vi "CleanUp fp settings.vi"(4 "Original basic fp settings":T1, 5 "Front Panel Window:Panel Bounds":T2, 6 "error in (no error)":errorcluster, 9 "vi reference":refnum<vi>) -> (0 "error out":errorcluster, 3 "vi reference out":refnum<vi>)   [LabVIEW 2020]
uses:
  <vilib>/Utility/miscctls.llb/LVRectTypeDef.ctl
  Basic FP Settings--cluster.ctl
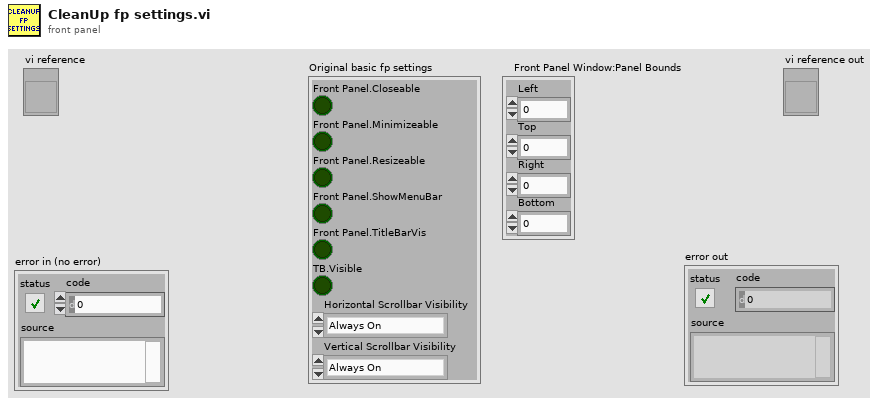
[diagram p1: front panel]
types:
  T1 = typedef "Basic FP Settings--cluster.ctl" = cluster{"Front Panel.Closeable":bool, "Front Panel.Minimizeable":bool, "Front Panel.Resizeable":bool, "Front Panel.ShowMenuBar":bool, "Front Panel.TitleBarVis":bool, "TB.Visible":bool, "Horizontal Scrollbar Visibility":enum16{"Always On", "Always Off", "Off While Running"}, "Vertical Scrollbar Visibility":enum16{"Always On", "Always Off", "Off While Running"}}
  T2 = typedef "LVRectTypeDef.ctl" = cluster{"Left":i16, "Top":i16, "Right":i16, "Bottom":i16}
  T3 = enum32{"Invalid", "Default", "Floating", "Floating/Auto-Hide", "Modal"}
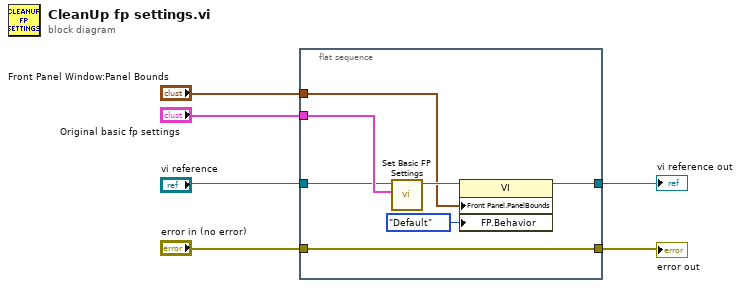
[diagram p0: block diagram]
diagram:
  n1 = flat-sequence {
    tunnel: "Original basic fp settings" -> [w11]
    tunnel: "Front Panel Window:Panel Bounds" -> [w10]
    tunnel: [w9] -> w6
    tunnel: "error in (no error)" -> [w9]
    tunnel: [w8] -> w5
    tunnel: "vi reference" -> [w7]
    frame #0 {
      n2 = call "Set Basic FP Settings.vi"("basic fp settings"=w11, "vi reference"=w7) -> ("vi reference out"=w13:refnum<vi>)  [unwired: 8 in, 1 out]
      n3 = property class="VI"(reference=w13, "Front Panel.PanelBounds"=w10, "FP.Behavior"=T3."Default" ("Front Panel Window:Behavior")) -> (reference out=w8:refnum<vi>)  [unwired: 1 in, 1 out]
    }
  }
  "error out" <- w6
  "vi reference out" <- w5
